vi "_Object Tester.vi"() -> ()   [LabVIEW 2025, in "Solenoid.lvclass"]
uses:
  Solenoid.lvclass
  Solenoid Selector.ctl
  EVI 79/EVI 79.lvclass
  C:/Users/grove/Desktop/LabVIEW/Git/atp-station/Classes/Solenoid/Solenoid.lvclass
  <vilib>/Handler Framework/Handler Framework.lvlib
panel:
  out "Wear_in":T1={"V"=24.0, "I"=0.5, "Cycles"=0.5, "On_Time_ms"=0.5, "Off_Time_ms"=0.5}
  out "Solenoid out":refnum<class "Solenoid.lvclass">
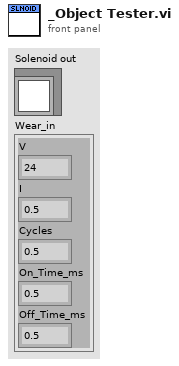
[diagram p1: front panel]
types:
  T1 = cluster{"V":dbl, "I":dbl, "Cycles":dbl, "On_Time_ms":dbl, "Off_Time_ms":dbl}
  T2 = typedef "Solenoid Selector.ctl" = enum16{"Generic Solenoid", "EVI-79"}
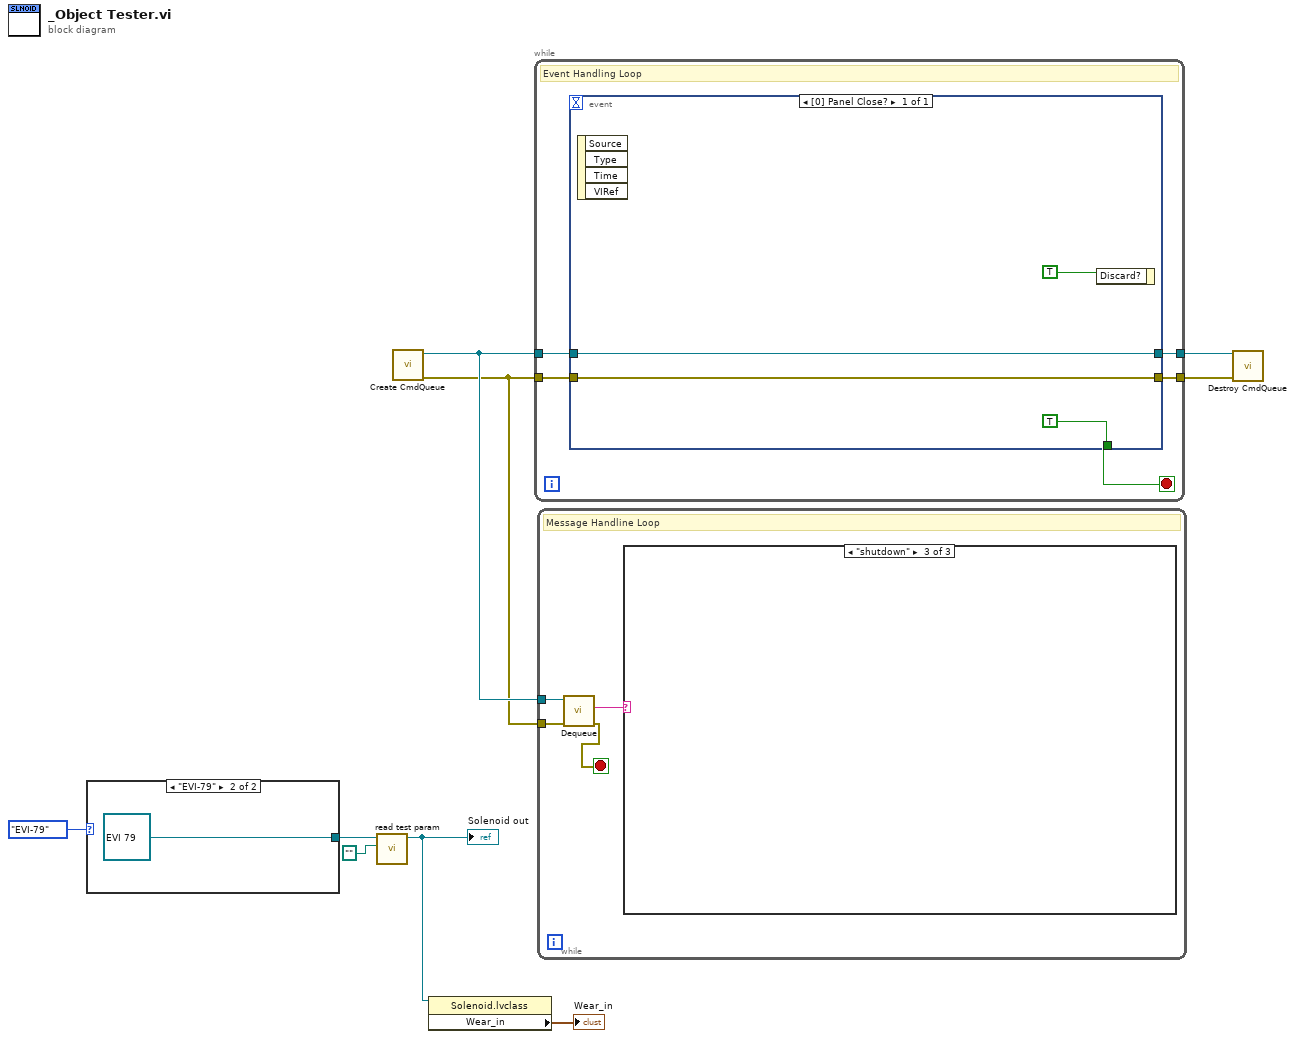
[diagram p0: block diagram]
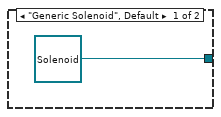
[diagram p2: hidden frame]
diagram:
  n1 = case shown="\"EVI-79\"" Solenoid_Selector."EVI-79" {
    tunnel: [refnum<class "Solenoid.lvclass"> refnum ("Solenoid.lvclass") refnum<class "EVI 79.lvclass"> refnum ("EVI 79.lvclass")] -> w4
    frame "Generic Solenoid", Default {
    }
    frame "EVI-79" {
    }
  }
  n2 = call-dynamic "read test param.vi"("File Path"=path "", "Solenoid in"=w4) -> ("Solenoid out"=w2:refnum<class "Solenoid.lvclass">)  [unwired: 8 in, 1 out]
  "Solenoid out" <- w2
  n3 = call <vilib>:"Create CmdQueue.vi"() -> ("error out"=w8:errorcluster, "CmdQueue out"=w9:refnum<queue>)  [unwired: 10 in]
  n4 = property class="Solenoid.lvclass"(reference=w2) -> ("Wear_in"=→"Wear_in":T1)  [unwired: 1 in, 2 out]
  n5 = while {
    tunnel: w9 -> [w15]
    tunnel: w8 -> [w14]
    tunnel: [w13] -> w7
    tunnel: [w12] -> w6
    stop <- w16 stop-if-true
    # "Event Handling Loop"
    n6 = event shown="[0] Panel Close?" {
      selector: _ -> [_]
      dyn-events: _ -> [_]
      timeout: _ -> [_]
      tunnel: [TRUE] -> w16
      tunnel: w15 -> [w18]
      tunnel: w14 -> [w17]
      tunnel: [w18] -> w13
      tunnel: [w17] -> w12
      event Panel Close? {
        n7 = event-data() -> ()  [unwired: 1 in, 4 out]
        n8 = event-data("Discard?"=TRUE) -> ()  [unwired: 1 in, 1 out]
      }
    }
  }
  n9 = while {
    tunnel: w9 -> [w24]
    tunnel: w8 -> [w23]
    stop <- w22 stop-if-true
    # "Message Handline Loop"
    n10 = call <vilib>:"Dequeue.vi"("error in (no error)"=w23, "CmdQueue in"=w24) -> ("error out"=w22:errorcluster, "cmd"=w21:string)  [unwired: 5 in, 3 out]
    n11 = case shown="\"shutdown\"" w21 {
      frame Default {
      }
      frame "init" {
      }
      frame "shutdown" {
      }
    }
  }
  n12 = call <vilib>:"Destroy CmdQueue.vi"("error in (no error)"=w6, "CmdQueue in"=w7) -> ()  [unwired: 9 in, 1 out]
